vi "response.From JSON Tree.vi"(8 "error in (no error)":errorcluster, 10 "JSON Value in":variant, 11 "Response in":refnum<class "Response.lvclass">) -> (0 "error out":errorcluster, 3 "Response out":refnum<class "Response.lvclass">)   [LabVIEW 2020, in "JSON-RPC Lib.lvlib" / "Response.lvclass"]
uses:
  Response.lvclass
  id/id.lvclass
  error/error.lvclass
  result/result.lvclass
  Response.lvclass/Response.ctl
  Variant Data Manipulation/Variant Data Manipulation.lvlib
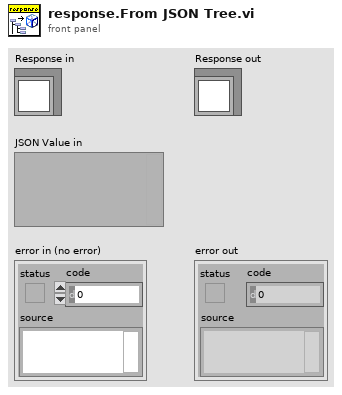
[diagram p1: front panel]
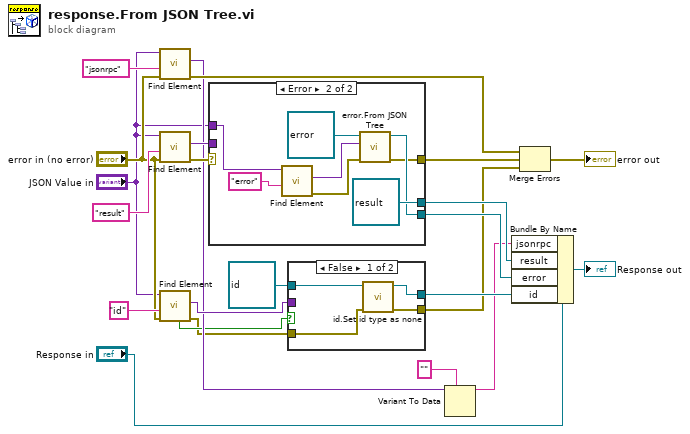
[diagram p0: block diagram]
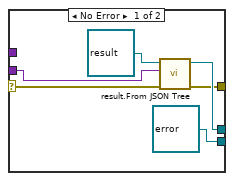
[diagram p2: hidden frame]
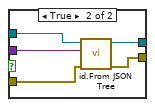
[diagram p3: hidden frame]
diagram:
  n1 = call "Find Element.vi"("error in (no error)"="error in (no error)", "Name"="jsonrpc" ("Parameter Name"), "Variant (Cluster) in"="JSON Value in") -> ("error out"=w12:errorcluster, "element"=w6:variant)  [unwired: 4 in, 3 out]
  n2 = call "Find Element.vi"("error in (no error)"="error in (no error)", "Name"="result" ("Parameter Name"), "Variant (Cluster) in"="JSON Value in") -> ("error out"=w10:errorcluster, "element"=w15:variant)  [unwired: 4 in, 3 out]
  n3 = call "Find Element.vi"("error in (no error)"="error in (no error)", "Name"="id" ("Parameter Name"), "Variant (Cluster) in"="JSON Value in") -> ("error out"=w1:errorcluster, "element"=w7:variant, "found?"=w2:bool)  [unwired: 4 in, 2 out]
  n4 = case shown="Error" w10 {
    selector: w10 -> [w25 _]
    tunnel: w15 -> [w24 _]
    tunnel: [w29 refnum<class "result.lvclass"> refnum ("result out")] -> w14
    tunnel: [refnum<class "error.lvclass"> refnum ("error") w34] -> w13
    tunnel: "JSON Value in" -> [_ w36]
    tunnel: [w26 w31] -> w11
    frame No Error {
      n5 = call "result.From JSON Tree.vi"("error in (no error)"=w25, "JSON Value in"=w24, "result in"=refnum<class "result.lvclass"> refnum) -> ("error out"=w26:errorcluster, "result out"=w29:refnum<class "result.lvclass">)  [unwired: 7 in]
    }
    frame Error {
      n6 = call "Find Element.vi"("Name"="error" ("key"), "Variant (Cluster) in"=w36) -> ("error out"=w32:errorcluster, "element"=w30:variant)  [unwired: 5 in, 3 out]
      n7 = call "error.From JSON Tree.vi"("error in (no error)"=w32, "JSON Value in"=w30, "error in"=refnum<class "error.lvclass"> refnum) -> (0:"error out"=w31:errorcluster, 3:"error out"=w34:refnum<class "error.lvclass">)  [unwired: 7 in]
    }
  }
  n8 = case shown="False" w2 {
    tunnel: refnum<class "id.lvclass"> refnum ("id.lvclass") -> [w41 w46]
    tunnel: [w40 w45] -> w19
    tunnel: [w39 w44] -> w9
    tunnel: w7 -> [_ w43]
    tunnel: w1 -> [w38 w42]
    frame False {
      n9 = call "id.Set id type as none.vi"("error in (no error)"=w38, "id in"=w41) -> ("error out"=w39:errorcluster, "id out"=w40:refnum<class "id.lvclass">)  [unwired: 8 in]
    }
    frame True {
      n10 = call "id.From JSON Tree.vi"("error in (no error)"=w42, "JSON Value in"=w43, "id in"=w46) -> ("error out"=w44:errorcluster, "id out"=w45:refnum<class "id.lvclass">)  [unwired: 7 in]
    }
  }
  n11 = Variant To Data(type="" ("Parameter Name"), Variant=w6) -> (data=w3:string)  [unwired: 1 in, 1 out]
  n12 = Bundle By Name(cluster="Response in", "jsonrpc"=w3, "result"=w14, "error"=w13, "id"=w19) -> (→"Response out":refnum<class "Response.lvclass">)
  n13 = Merge Errors(w12, w11, w9) -> (→"error out":errorcluster)
